vi "Test Assert String Not Starts With.vi"(8 "error in (no error)":errorcluster) -> (0 "error out":errorcluster)   [LabVIEW 2013]
uses:
  classes/Test/Test.lvclass
  classes/Assert/Assert.lvclass
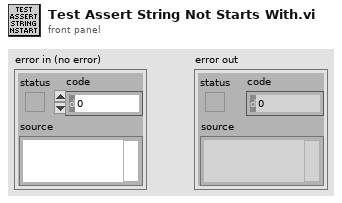
[diagram p1: front panel]
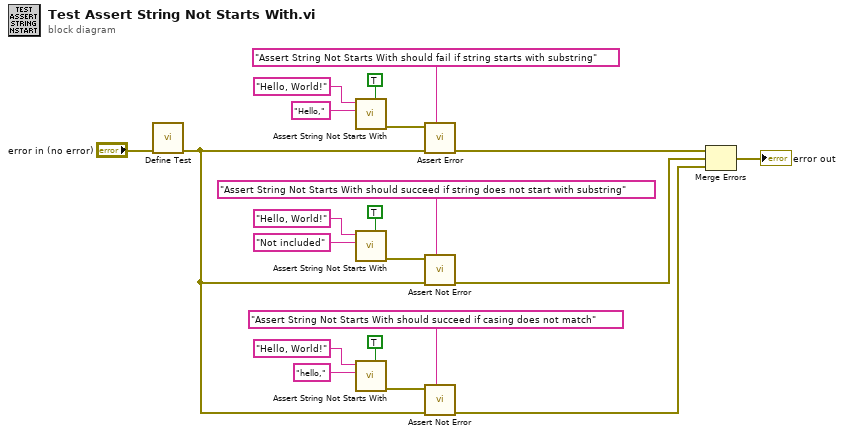
[diagram p0: block diagram]
diagram:
  n1 = call "Define Test.vi"("error in (no error)"="error in (no error)") -> ("error out"=w2:errorcluster)  [unwired: 9 in, 1 out]
  n2 = call "Assert String Not Starts With.vi"("Assert Only? (F)"=TRUE, "Substring"="Hello,", "String"="Hello, World!") -> ("error out"=w21:errorcluster)  [unwired: 7 in, 1 out]
  n3 = call "Assert String Not Starts With.vi"("Assert Only? (F)"=TRUE, "Substring"="Not included", "String"="Hello, World!") -> ("error out"=w9:errorcluster)  [unwired: 7 in, 1 out]
  n4 = call "Assert String Not Starts With.vi"("Assert Only? (F)"=TRUE, "Substring"="hello,", "String"="Hello, World!") -> ("error out"=w7:errorcluster)  [unwired: 7 in, 1 out]
  n5 = call "Assert Error.vi"("Label"="Assert String Not Starts With should fail if string starts with substring", "error in (no error)"=w2, "Error?"=w21) -> ("error out"=w17:errorcluster)  [unwired: 7 in, 1 out]
  n6 = call "Assert Not Error.vi"("Label"="Assert String Not Starts With should succeed if string does not start with substring", "error in (no error)"=w2, "Not Error?"=w9) -> ("error out"=w8:errorcluster)  [unwired: 7 in, 1 out]
  n7 = call "Assert Not Error.vi"("Label"="Assert String Not Starts With should succeed if casing does not match", "error in (no error)"=w2, "Not Error?"=w7) -> ("error out"=w1:errorcluster)  [unwired: 7 in, 1 out]
  n8 = Merge Errors(w17, w8, w1) -> (→"error out":errorcluster)
